vi "convert sonde cluster to spreadsheet array.vi"(10 "Cluster":T1 {"Salinity"."%" format="%_2f%%"; "Salinity"."Value" format="%_4g"; "Temperature"."%" format="%_2f%%"; "Temperature"."Value" format="%_4g"; "ORP"."%" format="%_2f%%"; "ORP"."Value" format="%_4g"; "pH"."%" format="%_2f%%"; "pH"."Value" format="%_4g"; "Dissolved Oxygen"."%" format="%_2f%%"; "Dissolved Oxygen"."Value" format="%_4g"; "Sp. Conductance"."%" format="%_2f%%"; "Sp. Conductance"."Value" format="%_4g"; "Cumulative\nVolume" format="%#_4g"}, 11 "Sheet":dbl) -> (1 "Time":string, 2 "Sonde Data Array from Cluster":dbl[](array[numeric]), 3 "sonde labels":string[](array[string])=["Sheet", "Final Reading (1=True)", "Final Tolerance (1=True)", "Head", "Depth", "Time seconds since 1Jan1904", "Cumulative Volume", "Sp. Cond. Value", "Sp. Cond. %", "Sp. Cond. Tolerance (1=True)", "DO Value", "DO %", "DO Tolerance (1=True)", "pH Value", "pH %", "pH Tolerance (1=True)", "ORP Value", "ORP %", "ORP Tolerance (1=True)", "Temp Value", "Temp %", "Temp. Tolerance (1=True)", "Salinity Value", "Salinity %", "Salinity Tolerance (1=True)", "Aux 1", "Aux 2", "Aux 3", "Time (HH:MM:SS)"], 5 "Sonde Data Array (String)":string[](array[string]))   [LabVIEW 2016]
uses:
  activeXtest/activeXtest 2015 Folder/sonde cluster from excel.ctl
  sdi_12/Sonde Value Percent Tol.ctl
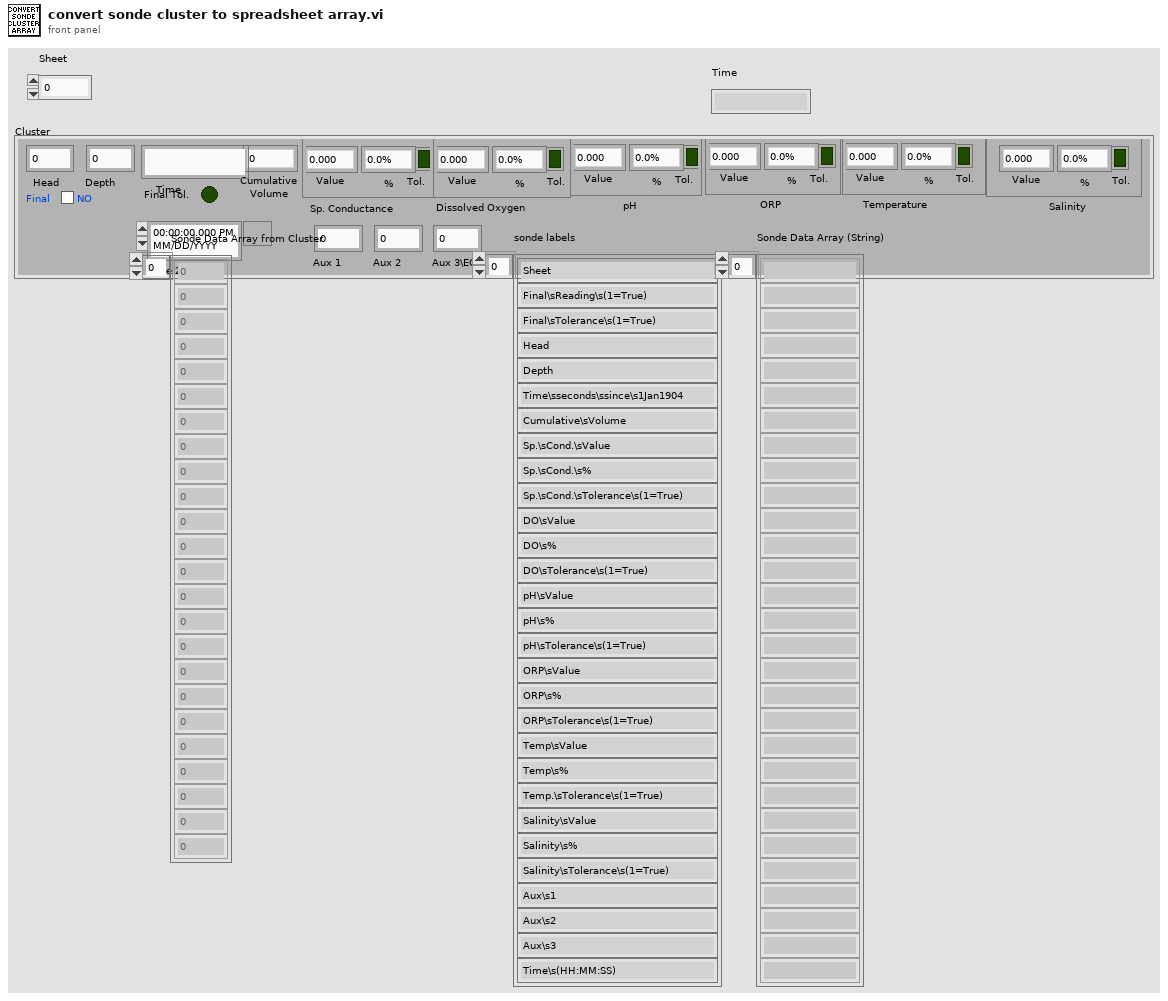
[diagram p1: front panel]
types:
  T1 = typedef "sonde cluster from excel.ctl" = cluster{"Head":dbl, "Depth":dbl, "Time":string, "Cumulative\nVolume":dbl, "Sp. Conductance":T2, "Dissolved Oxygen":T2, "pH":T2, "ORP":T2, "Temperature":T2, "Salinity":T2, "Final Tol.":bool, "Final":bool, "Time 2":timestamp, "Aux 1":dbl, "Aux 2":dbl, "Aux 3\\EC":dbl}
  T2 = typedef "Sonde Value Percent Tol.ctl" = cluster{"Value":dbl, "%":dbl, "Tol.":bool}
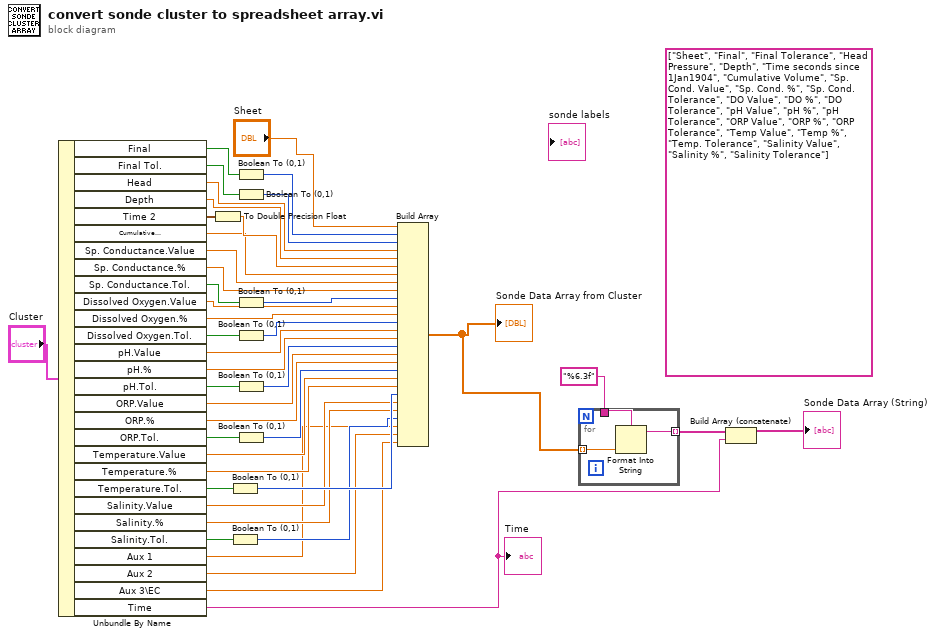
[diagram p0: block diagram]
diagram:
  (unwired) string[] ["Sheet", "Final", "Final Tolerance", "Head Pressure", "Depth", "Time seconds since 1Jan1904", "Cumulative Volume", "Sp. Cond. Value", "Sp. Cond. %", "Sp. Cond. Tolerance", "DO Value", "DO %", "DO Tolerance", "pH Value", "pH %", "pH Tolerance", "ORP Value", "ORP %", "ORP Tolerance", "Temp Value", "Temp %", "Temp. Tolerance", "Salinity Value", "Salinity %", "Salinity Tolerance"] ("sonde labels 2")
  n1 = Unbundle By Name("Cluster") -> ("Final"=w42:bool, "Final Tol."=w41:bool, "Head"=w5:dbl, "Depth"=w4:dbl, "Time 2"=w17:timestamp, "Cumulative\nVolume"=w2:dbl, "Sp. Conductance.Value"=w1:dbl, "Sp. Conductance.%"=w34:dbl, "Sp. Conductance.Tol."=w40:bool, "Dissolved Oxygen.Value"=w32:dbl, "Dissolved Oxygen.%"=w31:dbl, "Dissolved Oxygen.Tol."=w39:bool, "pH.Value"=w29:dbl, "pH.%"=w28:dbl, "pH.Tol."=w38:bool, "ORP.Value"=w26:dbl, "ORP.%"=w25:dbl, "ORP.Tol."=w37:bool, "Temperature.Value"=w23:dbl, "Temperature.%"=w22:dbl, "Temperature.Tol."=w36:bool, "Salinity.Value"=w20:dbl, "Salinity.%"=w19:dbl, "Salinity.Tol."=w35:bool, "Aux 1"=w16:dbl, "Aux 2"=w15:dbl, "Aux 3\\EC"=w14:dbl, "Time"=w9:string)
  "Time" <- w9
  n2 = To Double Precision Float(number=w17) -> (double precision float=w3:dbl)
  n3 = Boolean To (0,1)(Boolean=w36) -> (0, 1=w21:i16)
  n4 = Boolean To (0,1)(Boolean=w35) -> (0, 1=w18:i16)
  n5 = Boolean To (0,1)(Boolean=w42) -> (0, 1=w7:i16)
  n6 = Boolean To (0,1)(Boolean=w41) -> (0, 1=w6:i16)
  n7 = Boolean To (0,1)(Boolean=w40) -> (0, 1=w33:i16)
  n8 = Boolean To (0,1)(Boolean=w39) -> (0, 1=w30:i16)
  n9 = Boolean To (0,1)(Boolean=w38) -> (0, 1=w27:i16)
  n10 = Boolean To (0,1)(Boolean=w37) -> (0, 1=w24:i16)
  n11 = Build Array("Sheet", w7, w6, w5, w4, w3, w2, w1, w34, w33, w32, w31, w30, w29, w28, w27, w26, w25, w24, w23, w22, w21, w20, w19, w18, w16, w15, w14) -> (w13:dbl[])
  "Sonde Data Array from Cluster" <- w13
  n12 = for {
    tunnel: w13 -> [w46] mode=indexing
    tunnel: "%6.3f" ("format string") -> [w45]
    tunnel: [w44] -> w11 mode=indexing
    n13 = Format Into String(format string=w45, w46) -> (resulting string=w44:string)  [unwired: 2 in, 1 out]
  }
  n14 = Build Array (concatenate)(w11, w9) -> (→"Sonde Data Array (String)":string[])
